vi "fxpAverage.vi"(7 "reset":bool, 8 "doStep":bool, 11 "input":fxp<+/-,22,1>) -> (0 "dataValid":bool, 3 "averageOut":fxp<+/-,22,1>)   [LabVIEW 2016]
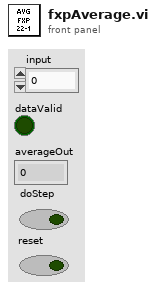
[diagram p1: front panel]
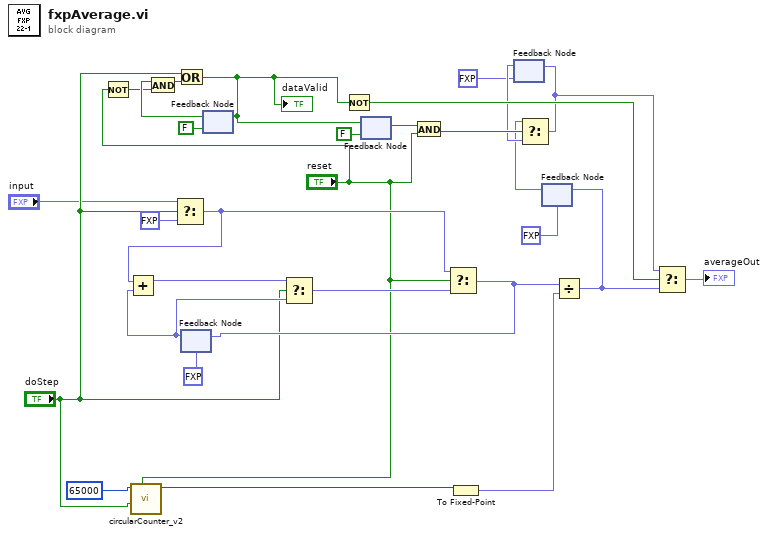
[diagram p0: block diagram]
diagram:
  n1 = Not(x="reset") -> (.not. x?=w21:bool)
  n2 = call "circularCounter_v2.vi"("reset"="reset", "doStep"="doStep", "maxCount"=u16 65000 ("countMax")) -> ("index"=w1:u16)  [unwired: 5 in, 3 out]
  n3 = Select(t="input", s="doStep", f=fxp<+/-,22,1> 0.0) -> (s? t:f=w20:fxp<+/-,22,1>)
  n4 = feedback #1(fxp<+/-,37,16> 0.0 ("f")) -> (w27:fxp<+/-,37,16>)
  n5 = Add(x=w20, y=w27) -> (x+y=w28:fxp<+/-,37,16>)
  n6 = feedback #2(FALSE) -> (w25:bool)
  n7 = And(x=w25, y=w21) -> (x .and. y?=w22:bool)
  n8 = Or(x="doStep", y=w22) -> (x .or. y?=w17:bool)
  "dataValid" <- w17
  n9 = feedback-in #2(w17) -> ()
  n10 = Select(t=w28, s="doStep", f=w27) -> (s? t:f=w29:fxp<+/-,37,16>)
  n11 = Not(x=w17) -> (.not. x?=w16:bool)
  n12 = feedback #3(FALSE) -> (w11:bool)
  n13 = feedback-in #3(w17) -> ()
  n14 = And(x=w11, y="reset") -> (x .and. y?=w24:bool)
  n15 = Select(t=w20, s="reset", f=w29) -> (s? t:f=w19:fxp<+/-,37,16>)
  n16 = feedback-in #1(w19) -> ()
  n17 = To Fixed-Point(number=w1) -> (fixed-point=w4:fxp<+,16,16>)  [unwired: 1 in]
  n18 = feedback #4(fxp<+/-,22,1> 0.0 ("f")) -> (w15:fxp<+/-,22,1>)
  n19 = feedback #5(fxp<+/-,22,1> 0.0 ("f")) -> (w12:fxp<+/-,22,1>)
  n20 = Select(t=w12, s=w24, f=w15) -> (s? t:f=w14:fxp<+/-,22,1>)
  n21 = feedback-in #4(w14) -> ()
  n22 = Divide(x=w19, y=w4) -> (x/y=w13:fxp<+/-,22,1>)
  n23 = feedback-in #5(w13) -> ()
  n24 = Select(t=w14, s=w16, f=w13) -> (s? t:f=→"averageOut":fxp<+/-,22,1>)
